vi "Read Next channel idx.vi"(8 "error in (no error)":errorcluster, 11 "Channel Scanner Driver in":refnum<class "Channel Scanner Driver.lvclass">) -> (0 "error out":errorcluster, 2 "Next channel idx":i32, 3 "Channel Scanner Driver out":refnum<class "Channel Scanner Driver.lvclass">)   [LabVIEW 2019, in "Channel Scanner Driver.lvclass"]
uses:
  Channel Scanner Driver.lvclass
  Channel Scanner Driver.lvclass/Channel Scanner Driver.ctl
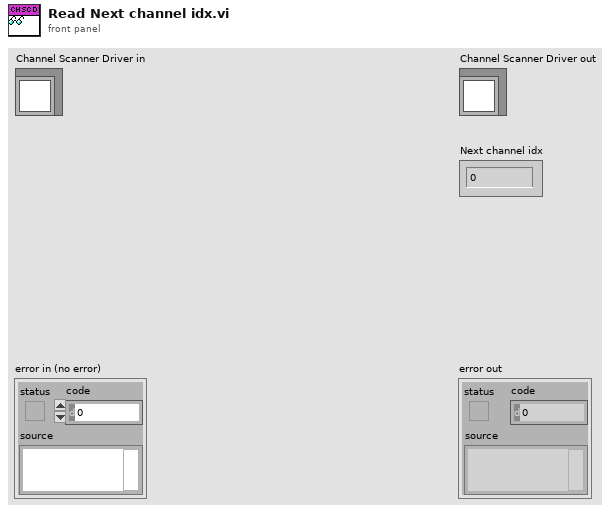
[diagram p1: front panel]
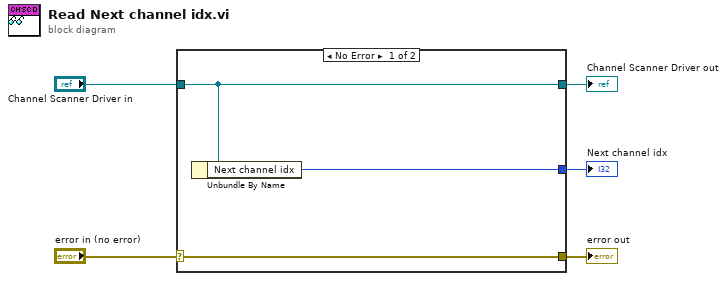
[diagram p0: block diagram]
diagram:
  n1 = case shown="No Error" "error in (no error)" {
    selector: "error in (no error)" -> [w8 w9]
    tunnel: [w8 w9] -> w4
    tunnel: [w7 w10] -> w2
    tunnel: "Channel Scanner Driver in" -> [w7 w10]
    tunnel: [w6 _] -> w1
    frame No Error {
      n2 = Unbundle By Name(w7) -> ("Next channel idx"=w6:i32)
    }
    frame Error {
    }
  }
  "error out" <- w4
  "Channel Scanner Driver out" <- w2
  "Next channel idx" <- w1
